vi "main_TSP.vi"() -> ()   [LabVIEW 2015]
uses:
  TSP Library/Class/TSP Class.lvclass
  <vilib>/event_ctls.llb/lveventtype.ctl
  TSP Library/TSP Library.lvlib
panel:
  out "Tour Best":u16[](array[numeric])
  out "Tour Opt":u16[](array[numeric])
  out "Distance Opt":dbl
  in  "Coordinate Load":bool
  in  "Mutation[%]":u8=5 min=1 max=100 step=5
  in  "ReInit":bool
  in  "Stop GA":bool
  in  "Delay":u32(slide)=100 scale=3.0..3000.0
  out "Distance":cluster{"Distance":dbl, "Distance":dbl}(graph)
  out "Distance Best":dbl
  out "Generation":u64
  in  "Start GA":bool
  in  "Create Population":bool
  in  "Coordinate RND":bool
  in  "Exit":bool
  in  "Size Best Save":u16=9
  in  "Size Population":u16=99
  out "City's":cluster{"X":dbl, "Y":dbl}[](graph)
  in  "City's":u16=13
  in  "Coordinate Min":dbl
  in  "Coordinate Max":dbl=100.0
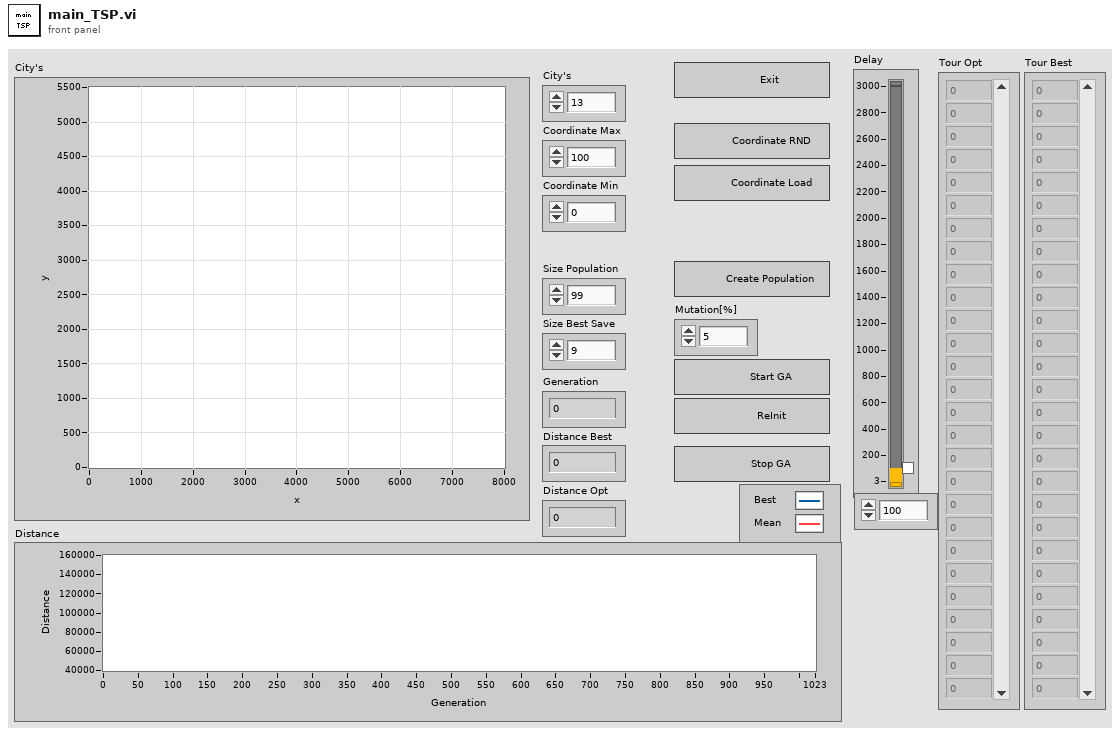
[diagram p1: front panel]
types:
  T1 = typedef "lveventtype.ctl" = enum32{"Null", "Timeout", "Annotation Menu Selection", "Annotation Menu Selection?", "App Instance Close", "App Instance Close?", "Autoscale Range Change", "Bookmark Info Change", "Cell Edit", "Cell Edit?", "Cursor Grab", "Cursor Grab?", "Cursor Menu Selection", "Cursor Menu Selection?", "Cursor Move", "Cursor Release", "Data Change", "Direction Change", "Display State Change", "Drag Ended", "Drag Enter", "Drag Leave", "Drag Over", "Drag Source Update", "Drag Starting", "Drag Starting?", "Drop", "Exec State Change", "Key Down", "Key Down?", "Key Repeat", "Key Repeat?", "Key Up", "Listbox Double Click", "Menu Activation?", "Menu Selection (App)", "Menu Selection? (App)", "Menu Selection (User)", "Mouse Down", "Mouse Down?", "Mouse Enter", "Mouse Leave", "Mouse Move", "Mouse Up", "Mouse Wheel", "NI Security User Change (App)", "Pane Size", "Panel Close", "Panel Close?", "Panel Resize", "Plot Attribute Change", "Scale Range Change", "Shortcut Menu Activation?", "Shortcut Menu Selection (App)", "Shortcut Menu Selection? (App)", "Shortcut Menu Selection (User)", "Tree Double Click", "Tree Drag", "Tree Drag?", "Tree Drop", "Tree Drop?", "Tree Item Close", "Tree Item Close?", "Tree Item Open", "Tree Item Open?", "User Event", "Value Change"}
  T2 = typedef "TSP Library.lvlib/Coordinate.ctl" = cluster{"x":dbl, "y":dbl}
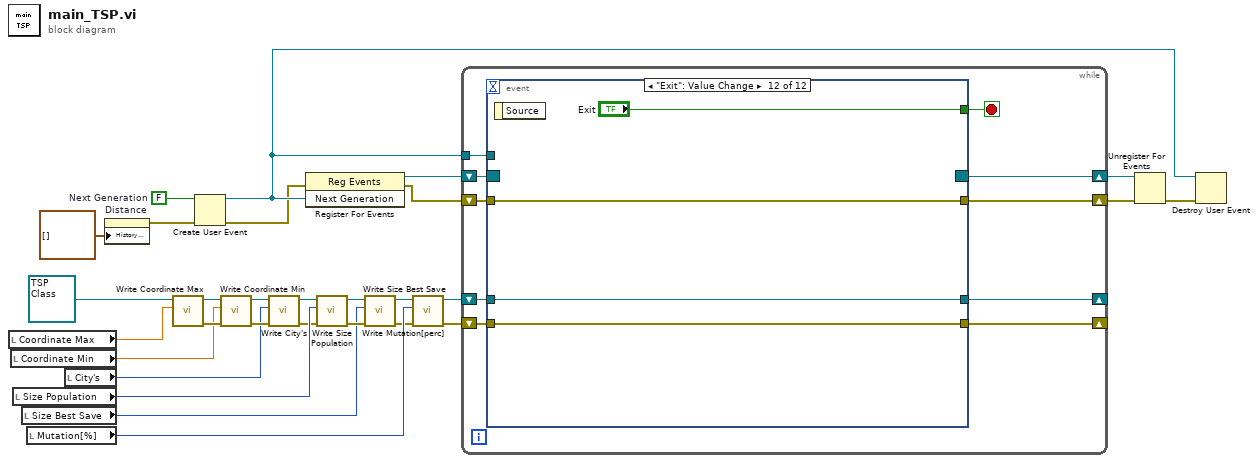
[diagram p0: block diagram]
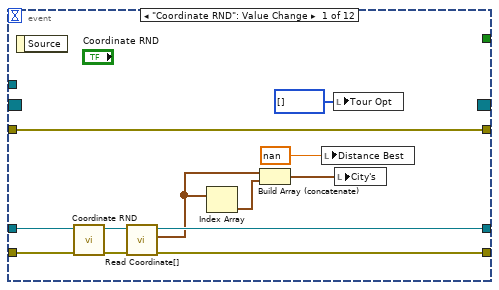
[diagram p2: hidden frame]
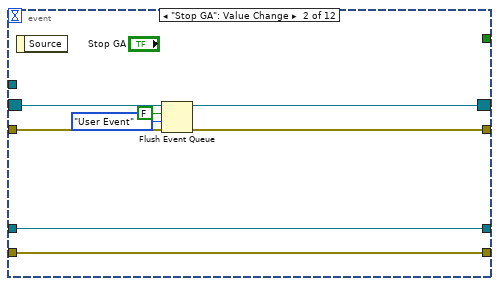
[diagram p3: hidden frame]
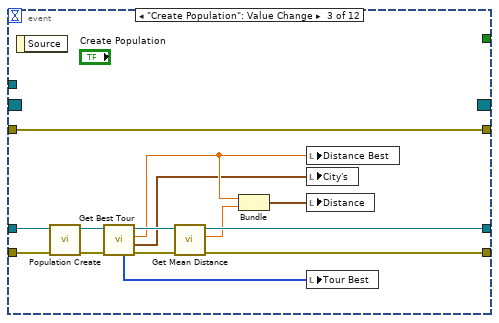
[diagram p4: hidden frame]
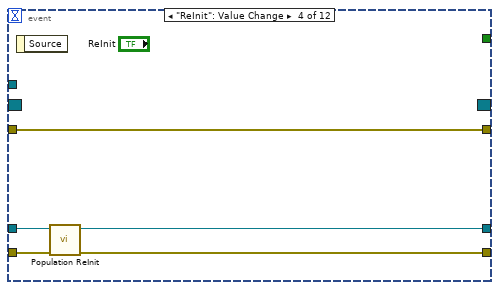
[diagram p5: hidden frame]
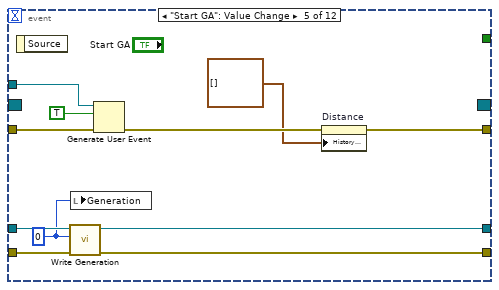
[diagram p6: hidden frame]
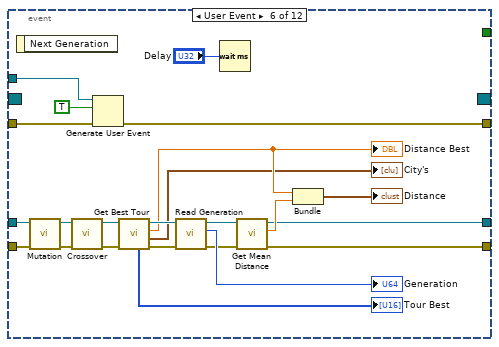
[diagram p7: hidden frame]
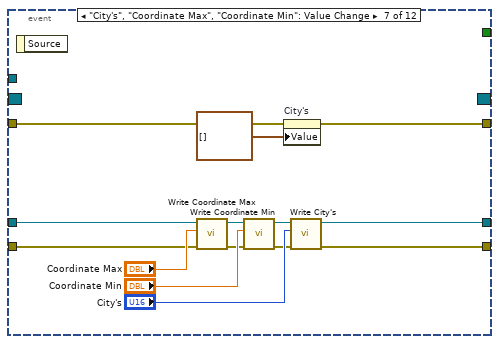
[diagram p8: hidden frame]
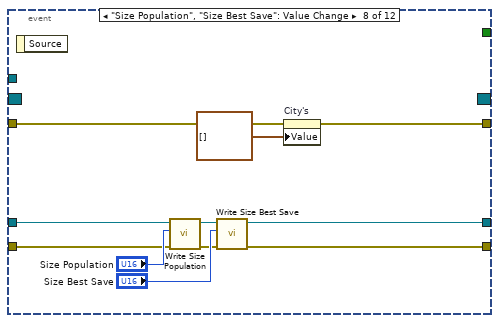
[diagram p9: hidden frame]
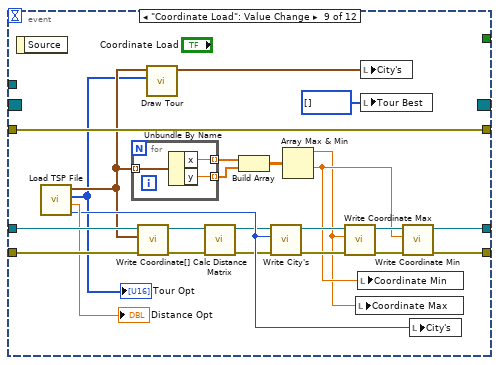
[diagram p10: hidden frame]
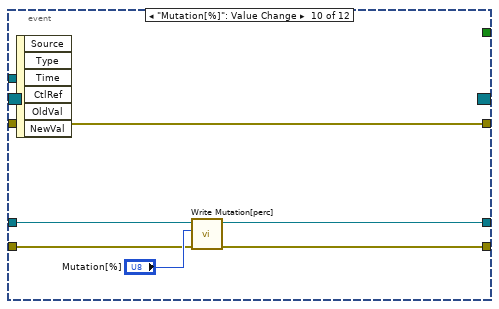
[diagram p11: hidden frame]
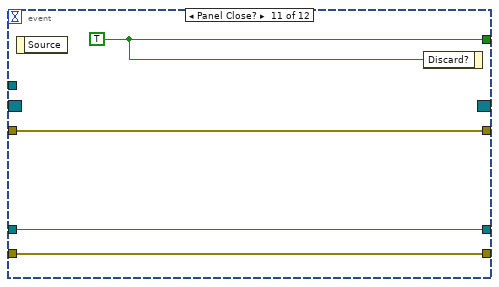
[diagram p12: hidden frame]
diagram:
  w29 = FALSE  # Next Generation
  n1 = local read "Coordinate Max"() -> (w3:dbl)
  n2 = local read "Coordinate Min"() -> (w2:dbl)
  n3 = local read "Size Population"() -> (w11:u16)
  n4 = local read "Size Best Save"() -> (w12:u16)
  n5 = local read "Mutation[%]"() -> (w17:u8)
  n6 = local read "City's"() -> (w1:u16)
  n7 = property on="Distance" class="WFChart (strict)"("History Data"=cluster{"Distance":dbl, "Distance":dbl}[] []) -> (error out=w23:errorcluster)  [unwired: 2 in, 1 out]
  n8 = call-dynamic "Write Coordinate Max.vi"("Coordinate Max"=w3, "TSP Class in"=refnum<class "TSP Class.lvclass"> refnum ("TSP Library:TSP Class.lvclass")) -> ("error out"=w8:errorcluster, "TSP Class out"=w10:refnum<class "TSP Class.lvclass">)  [unwired: 8 in]
  n9 = Create User Event(user event datatype=w29, error in=w23) -> (user event=w24:refnum<user-event>, error out=w20:errorcluster)
  n10 = call-dynamic "Write Coordinate Min.vi"("error in (no error)"=w8, "Coordinate Min"=w2, "TSP Class in"=w10) -> ("error out"=w7:errorcluster, "TSP Class out"=w9:refnum<class "TSP Class.lvclass">)  [unwired: 7 in]
  n11 = call-dynamic "Write City's.vi"("error in (no error)"=w7, "City's"=w1, "TSP Class in"=w9) -> ("error out"=w6:errorcluster, "TSP Class out"=w5:refnum<class "TSP Class.lvclass">)  [unwired: 7 in]
  n12 = register-events(error in=w20, w24) -> (reference out=w28:refnum<event-registration>, error out=w21:errorcluster)  [unwired: 1 in]
  n13 = call-dynamic "Write Size Population.vi"("error in (no error)"=w6, "Size Population"=w11, "TSP Class in"=w5) -> ("error out"=w15:errorcluster, "TSP Class out"=w16:refnum<class "TSP Class.lvclass">)  [unwired: 7 in]
  n14 = call-dynamic "Write Size Best Save.vi"("error in (no error)"=w15, "Size Best Save"=w12, "TSP Class in"=w16) -> ("error out"=w14:errorcluster, "TSP Class out"=w13:refnum<class "TSP Class.lvclass">)  [unwired: 7 in]
  n15 = call-dynamic "Write Mutation[perc].vi"("error in (no error)"=w14, "Mutation[%]"=w17, "TSP Class in"=w13) -> ("error out"=w19:errorcluster, "TSP Class out"=w18:refnum<class "TSP Class.lvclass">)  [unwired: 7 in]
  n16 = while {
    shift-right: [w37] -> _
    shift-left: w18 -> [w39]
    shift-right: [w36] -> _
    shift-left: w19 -> [w38]
    shift-right: [w33] -> w27
    shift-left: w28 -> [w34]
    shift-right: [w31] -> w26
    shift-left: w21 -> [w32]
    tunnel: w24 -> [w30]
    stop <- w35 stop-if-true
    n17 = event shown="[11] \"Exit\": Value Change" {
      selector: w34 -> [_ w57 _ _ _ _ _ _ _ _ _ _]
      dyn-events: [_ w56 _ _ _ _ _ _ _ _ _ _] -> w33
      timeout: _ -> [_ _ _ _ _ _ _ _ _ _ _ _]
      tunnel: w39 -> [w51 w53 w73 w78 w89 w106 w119 w133 w156 w168 w172 w176]
      tunnel: w38 -> [w50 w52 w72 w77 w88 w105 w118 w132 w160 w165 w171 w175]
      tunnel: [w47 w53 w67 w75 w80 w98 w117 w131 w153 w167 w172 w176] -> w37
      tunnel: [w46 w52 w66 w74 w79 w97 w116 w130 w157 w166 w171 w175] -> w36
      tunnel: [_ _ _ _ _ _ _ _ _ _ w174 "Exit"] -> w35
      tunnel: [w43 w58 w69 w76 w85 w111 w114 w127 w161 w170 w173 w177] -> w31
      tunnel: w32 -> [w43 w59 w69 w76 w86 w112 w115 w128 w161 w170 w173 w177]
      tunnel: w30 -> [_ _ _ _ w87 w110 _ _ _ _ _ _]
      event "Coordinate RND": Value Change {
        n18 = event-data() -> ()  [unwired: 1 in, 1 out]
        n19 = call-dynamic "Coordinate RND.vi"("error in (no error)"=w50, "TSP Class in"=w51) -> ("error out"=w48:errorcluster, "TSP Class out"=w49:refnum<class "TSP Class.lvclass">)  [unwired: 8 in]
        n20 = call-dynamic "Read Coordinate[].vi"("error in (no error)"=w48, "TSP Class in"=w49) -> ("error out"=w46:errorcluster, "Coordinate[]"=w44:T2[], "TSP Class out"=w47:refnum<class "TSP Class.lvclass">)  [unwired: 7 in]
        n21 = Index Array(array=w44) -> (element=w45:T2)  [unwired: 1 in]
        n22 = Build Array (concatenate)(w44, w45) -> (w41:T2[])
        n23 = local write "Distance Best"(nan ("Distance")) -> ()
        n24 = local write "Tour Opt"(u16[] [] ("Tour Opt")) -> ()
        n25 = local write "City's"(w41) -> ()
      }
      event "Stop GA": Value Change {
        n26 = event-data() -> ()  [unwired: 1 in, 1 out]
        n27 = Flush Event Queue(0:w57, 1:FALSE ("include static events? (T)"), 2:lveventtype."User Event" ("event type or object"), 3:w59) -> (8:w56:refnum<event-registration>, 11:w58:errorcluster)  [unwired: 2 in, 1 out]
      }
      event "Create Population": Value Change {
        n28 = event-data() -> ()  [unwired: 1 in, 1 out]
        n29 = call-dynamic "Population Create.vi"("error in (no error)"=w72, "TSP Class in"=w73) -> ("error out"=w70:errorcluster, "TSP Class out"=w71:refnum<class "TSP Class.lvclass">)  [unwired: 8 in]
        n30 = call-dynamic "Get Best Tour.vi"("error in (no error)"=w70, "TSP Class in"=w71) -> ("error out"=w65:errorcluster, "Coordinate[]"=w62:T2[], "Distance"=w63:dbl, "TSP Class out"=w68:refnum<class "TSP Class.lvclass">, "Tour"=w60:u16[])  [unwired: 5 in]
        n31 = call-dynamic "Get Mean Distance.vi"("error in (no error)"=w65, "TSP Class in"=w68) -> ("error out"=w66:errorcluster, "Distance Mean"=w64:dbl, "TSP Class out"=w67:refnum<class "TSP Class.lvclass">)  [unwired: 7 in]
        n32 = Bundle("Distance"=w63, "Distance Mean"=w64) -> (w61:cluster{"Distance":dbl, "Distance Mean":dbl})  [unwired: 1 in]
        n33 = local write "Distance Best"(w63) -> ()
        n34 = local write "City's"(w62) -> ()
        n35 = local write "Distance"(w61) -> ()
        n36 = local write "Tour Best"(w60) -> ()
      }
      event "ReInit": Value Change {
        n37 = event-data() -> ()  [unwired: 1 in, 1 out]
        n38 = call-dynamic "Population ReInit.vi"("error in (no error)"=w77, "TSP Class in"=w78) -> ("error out"=w74:errorcluster, "TSP Class out"=w75:refnum<class "TSP Class.lvclass">)  [unwired: 8 in]
      }
      event "Start GA": Value Change {
        w81 = u64 0 ("Generation")
        n39 = event-data() -> ()  [unwired: 1 in, 1 out]
        n40 = call-dynamic "Write Generation.vi"("error in (no error)"=w88, "Generation"=w81, "TSP Class in"=w89) -> ("error out"=w79:errorcluster, "TSP Class out"=w80:refnum<class "TSP Class.lvclass">)  [unwired: 7 in]
        n41 = local write "Generation"(w81) -> ()
        n42 = Generate User Event(user event=w87, event data cluster=TRUE ("event data"), error in=w86) -> (error out=w84:errorcluster)  [unwired: 1 in, 1 out]
        n43 = property on="Distance" class="WFChart (strict)"(error in=w84, "History Data"=cluster{"Distance":dbl, "Distance":dbl}[] []) -> (error out=w85:errorcluster)  [unwired: 1 in, 1 out]
      }
      event User Event {
        n44 = event-data() -> ()  [unwired: 1 in, 1 out]
        n45 = call-dynamic "Mutation.vi"("error in (no error)"=w105, "TSP Class in"=w106) -> ("error out"=w103:errorcluster, "TSP Class out"=w104:refnum<class "TSP Class.lvclass">)  [unwired: 8 in]
        n46 = call-dynamic "Crossover.vi"("error in (no error)"=w103, "TSP Class in"=w104) -> ("error out"=w95:errorcluster, "TSP Class out"=w94:refnum<class "TSP Class.lvclass">)  [unwired: 8 in]
        n47 = Generate User Event(user event=w110, event data cluster=TRUE ("event data"), error in=w112) -> (error out=w111:errorcluster)  [unwired: 1 in, 1 out]
        n48 = call-dynamic "Get Best Tour.vi"("error in (no error)"=w95, "TSP Class in"=w94) -> ("error out"=w108:errorcluster, "Coordinate[]"=→"City's":T2[], "Distance"=w93:dbl, "TSP Class out"=w109:refnum<class "TSP Class.lvclass">, "Tour"=→"Tour Best":u16[])  [unwired: 5 in]
        "Distance Best" <- w93
        n49 = call-dynamic "Read Generation.vi"("error in (no error)"=w108, "TSP Class in"=w109) -> ("error out"=w96:errorcluster, "Generation"=→"Generation":u64, "TSP Class out"=w99:refnum<class "TSP Class.lvclass">)  [unwired: 7 in]
        n50 = Wait (ms)(milliseconds to wait="Delay") -> ()  [unwired: 1 out]
        n51 = call-dynamic "Get Mean Distance.vi"("error in (no error)"=w96, "TSP Class in"=w99) -> ("error out"=w97:errorcluster, "Distance Mean"=w100:dbl, "TSP Class out"=w98:refnum<class "TSP Class.lvclass">)  [unwired: 7 in]
        n52 = Bundle("Distance"=w93, "Distance Mean"=w100) -> (→"Distance":cluster{"Distance":dbl, "Distance Mean":dbl})  [unwired: 1 in]
      }
      event "City's", "Coordinate Max", "Coordinate Min": Value Change {
        n53 = event-data() -> ()  [unwired: 1 in, 1 out]
        n54 = call-dynamic "Write Coordinate Max.vi"("error in (no error)"=w118, "Coordinate Max"="Coordinate Max", "TSP Class in"=w119) -> ("error out"=w122:errorcluster, "TSP Class out"=w120:refnum<class "TSP Class.lvclass">)  [unwired: 7 in]
        n55 = call-dynamic "Write Coordinate Min.vi"("error in (no error)"=w122, "Coordinate Min"="Coordinate Min", "TSP Class in"=w120) -> ("error out"=w123:errorcluster, "TSP Class out"=w121:refnum<class "TSP Class.lvclass">)  [unwired: 7 in]
        n56 = property on="City's" class="XYGraph (strict)"(error in=w115, "Value"=cluster{"X":dbl, "Y":dbl}[] [] ("City's")) -> (error out=w114:errorcluster)  [unwired: 1 in, 1 out]
        n57 = call-dynamic "Write City's.vi"("error in (no error)"=w123, "City's"="City's", "TSP Class in"=w121) -> ("error out"=w116:errorcluster, "TSP Class out"=w117:refnum<class "TSP Class.lvclass">)  [unwired: 7 in]
      }
      event "Size Population", "Size Best Save": Value Change {
        n58 = event-data() -> ()  [unwired: 1 in, 1 out]
        n59 = call-dynamic "Write Size Population.vi"("error in (no error)"=w132, "Size Population"="Size Population", "TSP Class in"=w133) -> ("error out"=w135:errorcluster, "TSP Class out"=w134:refnum<class "TSP Class.lvclass">)  [unwired: 7 in]
        n60 = call-dynamic "Write Size Best Save.vi"("error in (no error)"=w135, "Size Best Save"="Size Best Save", "TSP Class in"=w134) -> ("error out"=w130:errorcluster, "TSP Class out"=w131:refnum<class "TSP Class.lvclass">)  [unwired: 7 in]
        n61 = property on="City's" class="XYGraph (strict)"(error in=w128, "Value"=cluster{"X":dbl, "Y":dbl}[] [] ("City's")) -> (error out=w127:errorcluster)  [unwired: 1 in, 1 out]
      }
      event "Coordinate Load": Value Change {
        n62 = event-data() -> ()  [unwired: 1 in, 1 out]
        n63 = call "Load TSP File.vi"() -> ("DIMENSION"=w148:i32, "Distance Opt"=→"Distance Opt":dbl, "Tour Selection"=w139:i32[], "Coordinate[]"=w140:T2[])  [unwired: 8 in]
        "Tour Opt" <- w139
        n64 = for {
          tunnel: w140 -> [w164] mode=indexing
          tunnel: [w163] -> w152 mode=indexing
          tunnel: [w162] -> w151 mode=indexing
          n65 = Unbundle By Name(w164) -> ("x"=w163:dbl, "y"=w162:dbl)
        }
        n66 = call-dynamic "Write Coordinate[].vi"("error in (no error)"=w160, "Coordinate[]"=w140, "TSP Class in"=w156) -> ("error out"=w141:errorcluster, "TSP Class out"=w144:refnum<class "TSP Class.lvclass">)  [unwired: 7 in]
        n67 = call "Draw Tour.vi"("Tour"=w139, "Coordinate[]"=w140) -> ("City's"=w138:cluster{"X":dbl, "Y":dbl}[])  [unwired: 9 in]
        n68 = call-dynamic "Calc Distance Matrix.vi"("error in (no error)"=w141, "TSP Class in"=w144) -> ("error out"=w142:errorcluster, "TSP Class out"=w143:refnum<class "TSP Class.lvclass">)  [unwired: 8 in]
        n69 = Build Array(w152, w151) -> (w150:dbl[][])
        n70 = call-dynamic "Write City's.vi"("error in (no error)"=w142, "City's"=w148, "TSP Class in"=w143) -> ("error out"=w159:errorcluster, "TSP Class out"=w155:refnum<class "TSP Class.lvclass">)  [unwired: 7 in]
        n71 = Array Max & Min(array=w150) -> (max value=w146:dbl, min value=w147:dbl)  [unwired: 2 out]
        n72 = call-dynamic "Write Coordinate Max.vi"("error in (no error)"=w159, "Coordinate Max"=w146, "TSP Class in"=w155) -> ("error out"=w158:errorcluster, "TSP Class out"=w154:refnum<class "TSP Class.lvclass">)  [unwired: 7 in]
        n73 = local write "Coordinate Max"(w146) -> ()
        n74 = local write "Coordinate Min"(w147) -> ()
        n75 = local write "City's"(w138) -> ()
        n76 = local write "Tour Best"(u16[] [] ("Tour Best")) -> ()
        n77 = call-dynamic "Write Coordinate Min.vi"("error in (no error)"=w158, "Coordinate Min"=w147, "TSP Class in"=w154) -> ("error out"=w157:errorcluster, "TSP Class out"=w153:refnum<class "TSP Class.lvclass">)  [unwired: 7 in]
        n78 = local write "City's"(w148) -> ()
      }
      event "Mutation[%]": Value Change {
        n79 = event-data() -> ()  [unwired: 1 in, 6 out]
        n80 = call-dynamic "Write Mutation[perc].vi"("error in (no error)"=w165, "Mutation[%]"="Mutation[%]", "TSP Class in"=w168) -> ("error out"=w166:errorcluster, "TSP Class out"=w167:refnum<class "TSP Class.lvclass">)  [unwired: 7 in]
      }
      event Panel Close? {
        w174 = TRUE ("Exit")
        n81 = event-data() -> ()  [unwired: 1 in, 1 out]
        n82 = event-data("Discard?"=w174) -> ()  [unwired: 1 in, 1 out]
      }
      event "Exit": Value Change {
        n83 = event-data() -> ()  [unwired: 1 in, 1 out]
      }
    }
  }
  n84 = Unregister For Events(event registration refnum=w27, error in=w26) -> (error out=w25:errorcluster)
  n85 = Destroy User Event(user event=w24, error in=w25) -> ()  [unwired: 1 out]
